vi "Get Next Non-Text Sibling.vi"(8 "error in (no error)":errorcluster, 11 "node in":refnum<k20>) -> (0 "error out":errorcluster, 1 "found sibling node?":bool, 2 "sibling node":refnum<k20>, 3 "node out":refnum<k20>)   [LabVIEW 2020, in "NI_XML.lvlib"]
doc: "Returns the first sibling of the <B>node in</B> that is not of type <B>Text_Node</B>."
uses:
  <vilib>/xml/NI_XML.lvlib
  <vilib>/xml/Close Reference(Node).vi
  <resource>/objmgr/DOMUserDefRef.rc
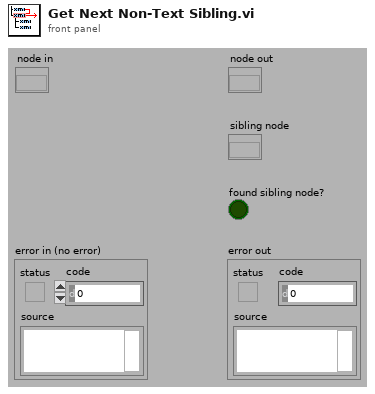
[diagram p1: front panel]
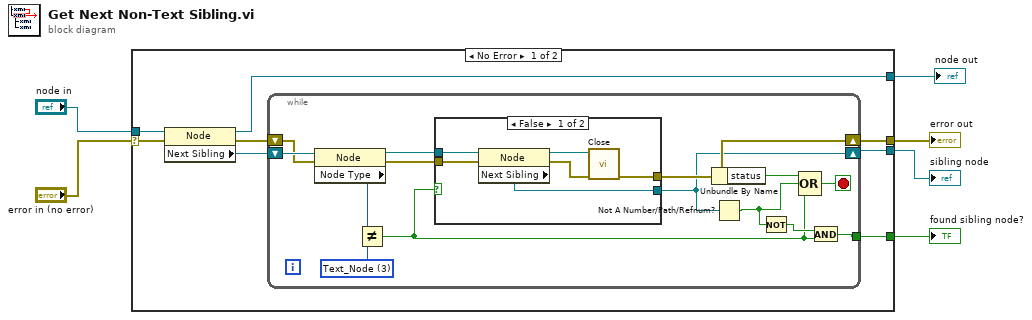
[diagram p0: block diagram]
diagram:
  n1 = case shown="No Error" "error in (no error)" {
    selector: "error in (no error)" -> [w7 w37]
    tunnel: "node in" -> [w14 w38]
    tunnel: [w11 w38] -> w5
    tunnel: [w10 w37] -> w4
    tunnel: [w9 _] -> w3
    tunnel: [w8 _] -> w2
    frame No Error {
      n2 = property class="Node"(reference=w14, error in=w7) -> (reference out=w11:refnum<k20>, error out=w12:errorcluster, "Next Sibling"=w13:refnum<k20>)
      n3 = while {
        shift-right: [w20] -> w9
        shift-left: w13 -> [w28]
        shift-right: [w22] -> w10
        shift-left: w12 -> [w27]
        tunnel: [w15] -> w8
        stop <- w24 stop-if-true
        w19 = 3 items=["Element_Node"=1, "Attribute_Node"=2, "Text_Node"=3, "CDATASection_Node"=4, "EntityReference_Node"=5, "Entity_Node"=6, "ProcessingInstruction_Node"=7, "Comment_Node"=8, "Document_Node"=9, "DocumentType_Node"=10, "DocumentFragment_Node"=11, "Notation_Node"=12] ("Node Type")
        n4 = property class="Node"(reference=w28, error in=w27) -> (reference out=w21:refnum<k20>, error out=w23:errorcluster, "Node Type"=w26:i32)
        n5 = Not Equal?(x=w26, y=w19) -> (x != y?=w16:bool)
        n6 = case shown="False" w16 {
          tunnel: w21 -> [w34 w35]
          tunnel: w23 -> [w33 w36]
          tunnel: [w29 w36] -> w22
          tunnel: [w31 w35] -> w20
          frame False {
            n7 = property class="Node"(reference=w34, error in=w33) -> (reference out=w32:refnum<k20>, error out=w30:errorcluster, "Next Sibling"=w31:refnum<k20>)
            n8 = call-poly <vilib>:"Close.vi"("error in (no error)"=w30, "node"=w32) -> ("error out"=w29:errorcluster)  [unwired: 7 out]
          }
          frame True {
          }
        }
        n9 = Unbundle By Name(w22) -> ("status"=w25:bool)
        n10 = Not A Number/Path/Refnum?(number/path/refnum=w20) -> (NaN/Path/Refnum?=w18:bool)
        n11 = Not(x=w18) -> (.not. x?=w17:bool)
        n12 = Compound Arithmetic op=OR(w25, w18, w16) -> (w24:bool)
        n13 = And(x=w17, y=w16) -> (x .and. y?=w15:bool)
      }
    }
    frame Error {
    }
  }
  "node out" <- w5
  "error out" <- w4
  "sibling node" <- w3
  "found sibling node?" <- w2
